vi "Analog Read Benchmark.vi"(0 "Stop Button":bool, 11 "AO Channels":u8[](array[numeric])=[0, 0, 0, 0, 0, 0, 0, 0, 0, 0, 0, 0]) -> (2 "Voltages":dbl[](array[numeric]), 3 "Loop Time (ms)":i32, 6 "Loop Rate":dbl(graph), 7 "Device Name":string)   [LabVIEW 2011]
uses:
  Private/Type Defs/Interface.ctl
  Private/Device/Device.lvlib
  LVH-LINX.lvlib
  <vilib>/ptbypt/NI_PtbyPt.lvlib
panel:
  out "Voltages":dbl[](graph)
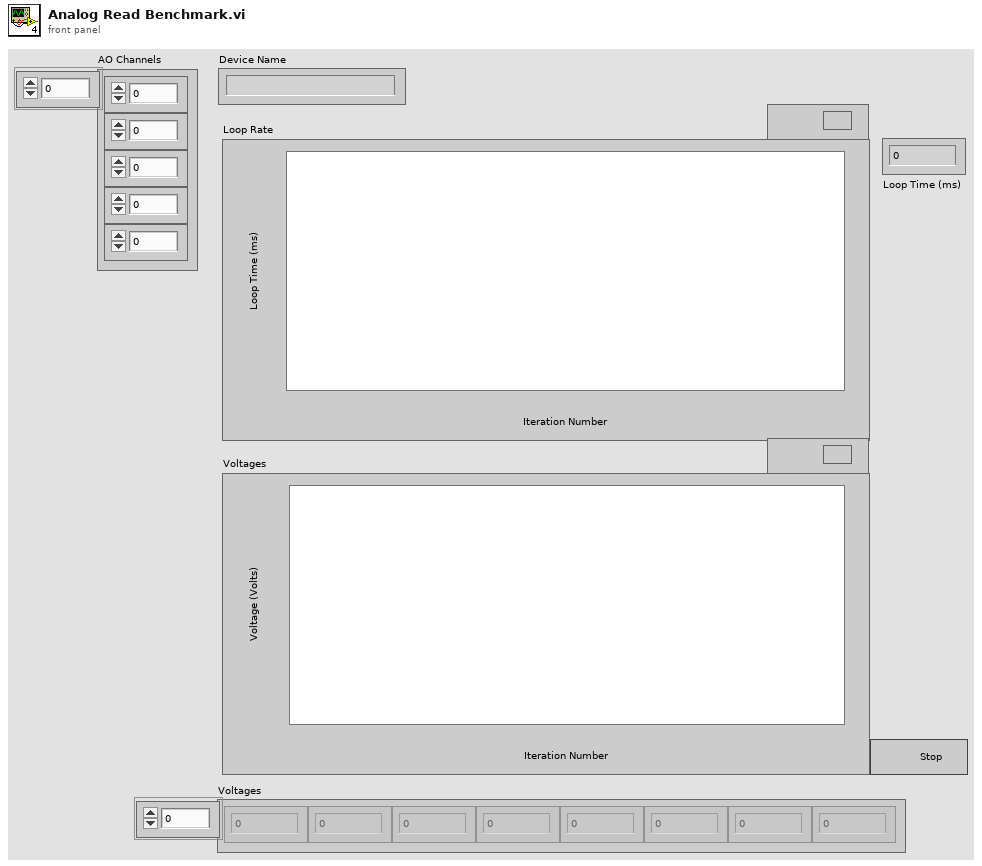
[diagram p1: front panel]
types:
  T1 = typedef "LVH-LINX.lvlib/Interface.ctl" = enum16{"Serial", "TCP"}
  T2 = typedef "LVH-LINX.lvlib/Device.lvlib/LINX Device Config.ctl" = cluster{"Interface":T1, "COM Port":refnum<visa-resource-name>, "TCP Configuration":T3, "Device Family":T4, "Device ID":u8, "Device Name":string, "TCP Ref":refnum<k5>}
  T3 = typedef "LVH-LINX.lvlib/Device.lvlib/TCP Config.ctl" = cluster{"IP Address":string, "Port":u16}
  T4 = typedef "LVH-LINX.lvlib/Device Family.ctl" = enum8{"National Instruments", "Digilent", "Arduino"}
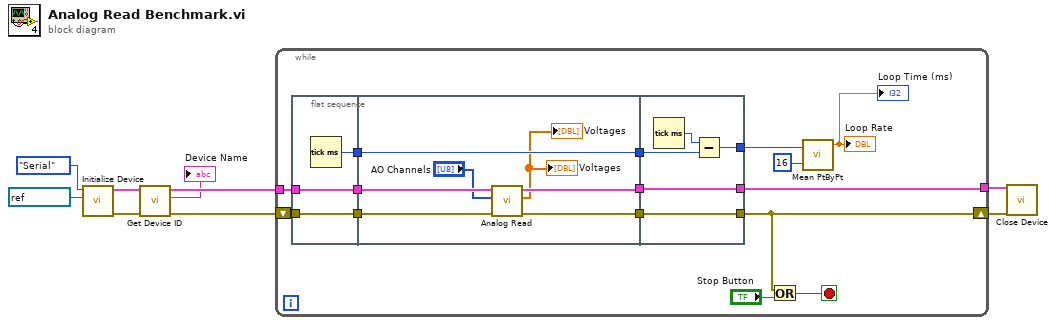
[diagram p0: block diagram]
diagram:
  n1 = call "Initialize Device.vi"("COM Port"=refnum<visa-resource-name> "COM5", "Interface"=Interface."Serial") -> ("Error Out"=w5:errorcluster, "LINX Device Config"=w6:T2)  [unwired: 8 in]
  n2 = call "Get Device ID.vi"("Error In"=w5, "LINX Device Config"=w6) -> ("Error Out"=w4:errorcluster, "Device Name"=→"Device Name":string, "LINX Device Config"=w3:T2)  [unwired: 7 in]
  n3 = while {
    tunnel: w3 -> [w24]
    shift-right: [w10] -> w7
    shift-left: w4 -> [w12]
    tunnel: [w15] -> w1
    stop <- w23 stop-if-true
    n4 = flat-sequence {
      tunnel: w24 -> [w27]
      tunnel: [w27] -> w21
      tunnel: [w26] -> w20
      tunnel: w12 -> [w25]
      tunnel: [w25] -> w11
      tunnel: w21 -> [w33]
      tunnel: w20 -> [w34]
      tunnel: [w34] -> w19
      tunnel: [w32] -> w14
      tunnel: [w31] -> w13
      tunnel: w11 -> [w30]
      tunnel: w19 -> [w38]
      tunnel: [w37] -> w18
      tunnel: [w36] -> w15
      tunnel: w14 -> [w36]
      tunnel: w13 -> [w35]
      tunnel: [w35] -> w10
      frame #0 {
        n5 = Tick Count (ms)() -> (millisecond timer value=w26:u32)
      }
      frame #1 {
        n6 = call "Analog Read.vi"("Error In"=w30, "AI Channels"="AO Channels", "LINX Device Config"=w33) -> ("Error Out"=w31:errorcluster, "Voltages"=→"Voltages" →"Voltages":dbl[], "LINX Device Config"=w32:T2)  [unwired: 6 in]
      }
      frame #2 {
        n7 = Tick Count (ms)() -> (millisecond timer value=w39:u32)
        n8 = Subtract(x=w39, y=w38) -> (x-y=w37:u32)
      }
    }
    n9 = Or(x=w10, y="Stop Button") -> (x .or. y?=w23:bool)
    n10 = call <vilib>:"Mean PtByPt.vi"("x"=w18, "sample length"=16) -> ("mean"=→"Loop Rate" →"Loop Time (ms)":dbl)  [unwired: 2 in, 1 out]
  }
  n11 = call "Close Device.vi"("Error In"=w7, "LINX Device Config"=w1) -> ()  [unwired: 8 in, 2 out]
